vi "Load Replay Data From CSV.vi"(5 "Memory Size as number":i32=32768, 6 "CycleAngle?":T1, 9 "MissingTeeth Location":dbl=200.0, 10 "ReverseData":bool, 11 "File Path":path=path "C:/Users/sbarrett/Documents/SVN/Engine Simulation/Engine Sim FPGA Example/crank VR data.csv") -> (0 "error out":errorcluster, 1 "Selected Length":i32, 2 "Selected Offset":i32, 3 "Data":dbl[](graph), 4 "DAC data":i16[](array[numeric]))   [LabVIEW 2013]
uses:
  Data File Loader/AngleReference.ctl
  Data File Loader/Data Replay Data Selection Method.ctl
  Data File Loader/Data Replay File.lvlib
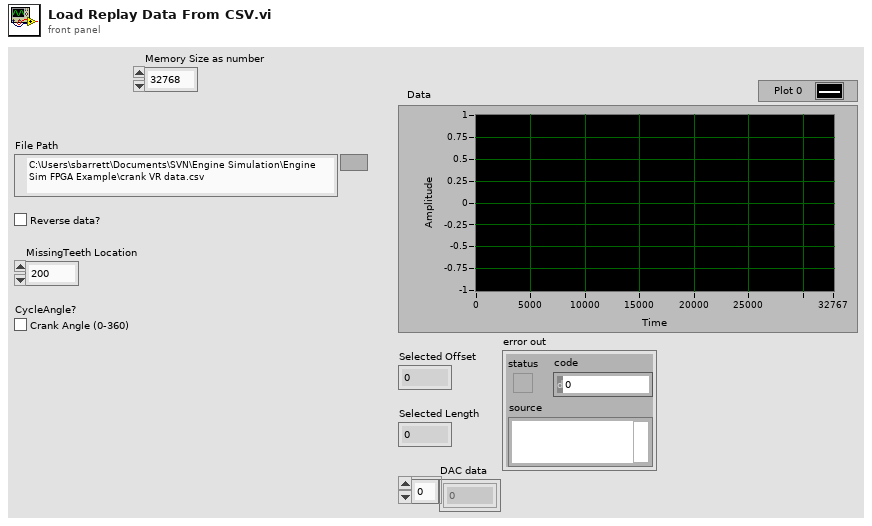
[diagram p1: front panel]
types:
  T1 = typedef "AngleReference.ctl" = bool
  T2 = typedef "Data Replay Data Selection Method.ctl" = enum32{"Manual", "AutoVRCrank"}
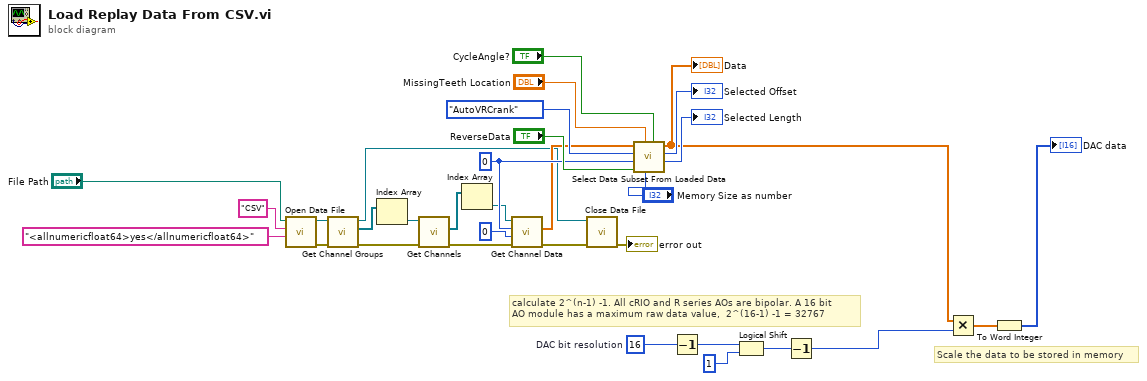
[diagram p0: block diagram]
diagram:
  w5 = u8 16  # DAC bit resolution
  w27 = 0 ("index")
  # "calculate 2^(n-1) -1. All cRIO and R series AOs are bipolar. A 16 bit\nAO module has a maximum raw data value,  2^(16-1) -1 = 32767"
  # "Scale the data to be stored in memory"
  n1 = call "Open Data File.vi"("Additional parameters"="<allnumericfloat64>yes</allnumericfloat64>" ("Data Plugin"), "Data Plugin"="CSV", "File Path"="File Path") -> ("error out"=w10:errorcluster, "File Ref"=w17:refnum<k20>)  [unwired: 7 in]
  n2 = call "Get Channel Groups.vi"("error in (no error)"=w10, "File Ref in"=w17) -> ("error out"=w11:errorcluster, "Channel Groups"=w19:refnum<k20>[], "File Ref out"=w18:refnum<k20>)  [unwired: 7 in]
  n3 = Index Array(array=w19) -> (element=w20:refnum<k20>)  [unwired: 1 in]
  n4 = call "Get Channels.vi"("error in (no error)"=w11, "Channel Group in"=w20) -> ("error out"=w12:errorcluster, "Channels"=w21:refnum<k20>[])  [unwired: 7 in, 1 out]
  n5 = Index Array(array=w21) -> (element=w22:refnum<k20>)  [unwired: 1 in]
  n6 = call "Get Channel Data.vi"("error in"=w12, "Count (0: Read All)"=0, "index"=w27, "Channel in"=w22) -> ("error out"=w13:errorcluster, "Signal"=w24:dbl[])  [unwired: 5 in, 1 out]
  n7 = call "Close Data File.vi"("error in (no error)"=w13, "File Ref"=w18) -> ("error out"=→"error out":errorcluster)  [unwired: 9 in]
  n8 = call "Select Data Subset From Loaded Data.vi"("CycleAngle?"="CycleAngle?", "Memory Size as number"="Memory Size as number", "MissingTeeth"="MissingTeeth Location", "ReverseData"="ReverseData", "Offset"=w27, "Data Selection Method"=Data_Replay_Data_Selection_Method."AutoVRCrank", "Signal"=w24) -> ("Selected Length"=→"Selected Length":i32, "Selected Offset"=→"Selected Offset":i32, "Resampled Data"=w2:dbl[])  [unwired: 2 in]
  "Data" <- w2
  n9 = Decrement(x=w5) -> (x-1=w7:u8)
  n10 = Logical Shift(y=w7, x=i16 1) -> (x << y=w8:i16)
  n11 = Decrement(x=w8) -> (x-1=w3:i16)
  n12 = Multiply(x=w2, y=w3) -> (x*y=w4:dbl[])
  n13 = To Word Integer(number=w4) -> (16bit integer=→"DAC data":i16[])
